vi "ConvertRefToDynamicAcq.vi"(10 "FPGA Ref":refnum<k20>) -> (2 "FPGA Ref":T1)   [LabVIEW 2017, in "cRIOWfmLib.lvlib"]
uses:
  <vilib>/addons/InsightCM/Devices/Shared/Cms/cRIOWfmAcq/cRIOWfmLib.lvlib
  <vilib>/addons/InsightCM/Devices/Shared/Cms/cRIOWfmAcq/subVIs/RIO Wfm Cust Ctrls/rwfm_DynamicFPGAref2.ctl
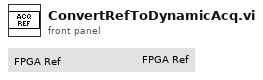
[diagram p1: front panel]
types:
  T1 = typedef "cRIOWfmLib.lvlib/rwfm_DynamicFPGAref2.ctl" = refnum<k20>
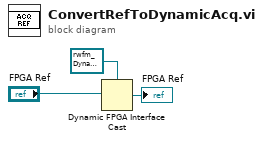
[diagram p0: block diagram]
diagram:
  n1 = Dynamic FPGA Interface Cast(Session In=T1 refnum ("Dynamic FPGA Ref"), Type="FPGA Ref") -> (Session Out=→"FPGA Ref":T1)
